vi "Read_Write_ADAM_setup.vi"(3 "Mode":T1(ring)) -> ()   [LabVIEW 2010]
uses:
  ADAM Client/Sub VIs/ADAM Controls/Channel_State.ctl
  Anemometry/Anemometry Sub Vis/Globals/Constants_global.vi
  Anemometry/Anemometry Sub Vis/Globals/Gas_management_global.vi
  Exp conditions/EnFlo_Tun_Setup_global.vi
  ADAM_Global.vi
  Channel_Description_Global.vi
panel:
  out "Setup Filename":string
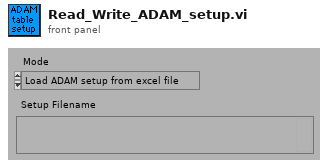
[diagram p1: front panel]
types:
  T1 = enum16{"Load ADAM setup from excel file", "Save ADAM setup to excel file"}
  T2 = typedef "Channel_State.ctl" = enum16{"On", "Off", "Always On", "Always Off"}
  T3 = typedef "Ch_description_ADAM.ctl" = cluster{"Ch Name":string, "Type":T4, "Function":T5, "Ch State":T2, "Calibration type":T6, "A":dbl, "B":dbl, "C":dbl, "D":dbl, "Comments":string, "Address":T7, "String":string, "Duty":u16}
  T4 = typedef "Module_type_ADAM.ctl" = enum16{"4011", "4012", "4013", "4014", "4016", "4017", "4018", "4021", "4050", "4052", "4053", "4060", "4080", "5000", "5017", "5018", "5024", "5051", "5056", "5060", "6060", "Tracker", "WEST", "GILL", "JEM", "VICI", "Vaisala", "DRUCK", "Run VI Named:", "IR2100", "PPT", "Comparator", "VIRTUAL", "Hold Value", "Read A", "Read Ch", "Coded", "Client Info", "Web Client", "X10", "Test"}
  T5 = typedef "Function_ADAM.ctl" = enum16{"Analogue Input", "Digital Input", "Event counter", "Event rate", "Analogue Output", "Digital Output", "Relay Output"}
  T6 = typedef "Calib_type_ADAM.ctl" = enum16{"Raw", "Bx + A", "Cx^2 + Bx + A", "Dx^3 + Cx^2 + Bx + A", "In Band", "Hi-Tec Q", "Hi-Tec M_dot", "Text"}
  T7 = typedef "Address.ctl" = cluster{"Main":i32, "Ch.":i32, "Sub":i32, "Port Name":string}
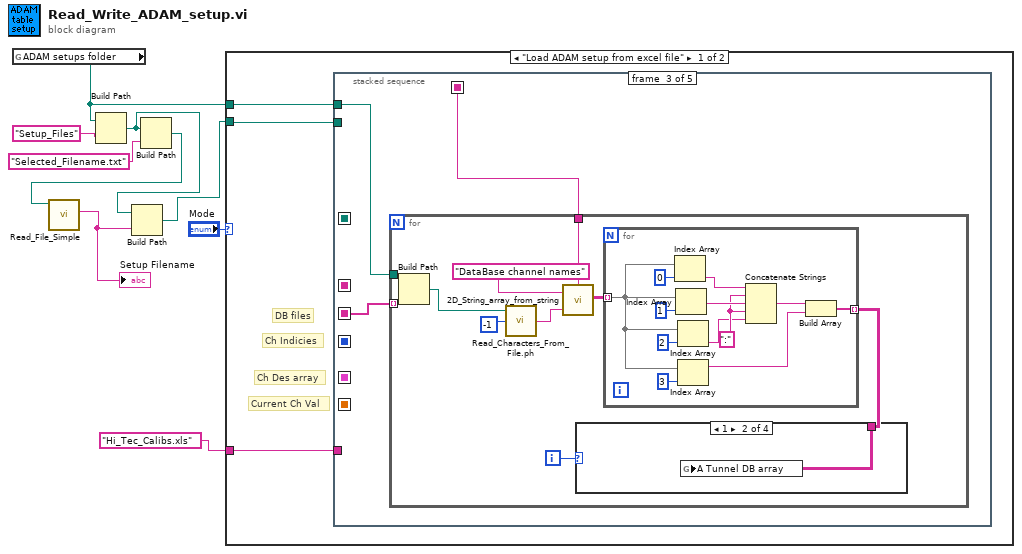
[diagram p0: block diagram]
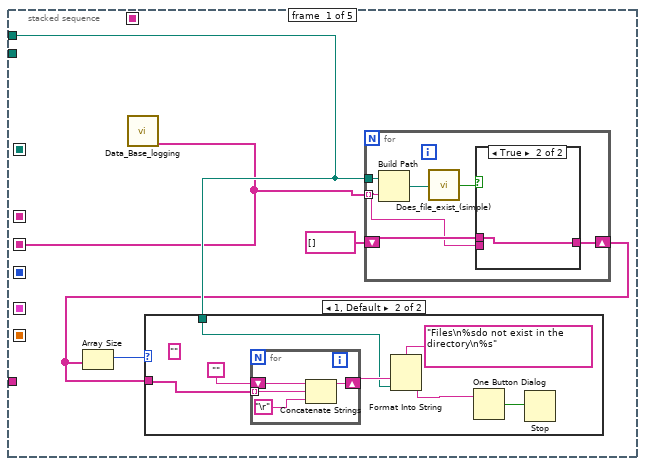
[diagram p2: hidden frame]
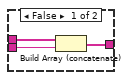
[diagram p4: hidden frame]
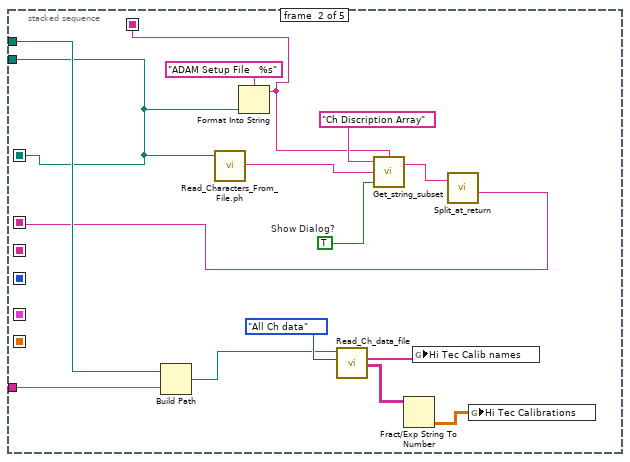
[diagram p5: hidden frame]
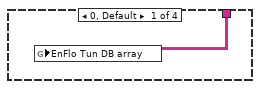
[diagram p6: hidden frame]
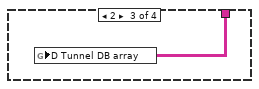
[diagram p7: hidden frame]
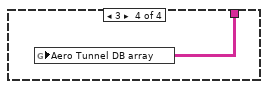
[diagram p8: hidden frame]
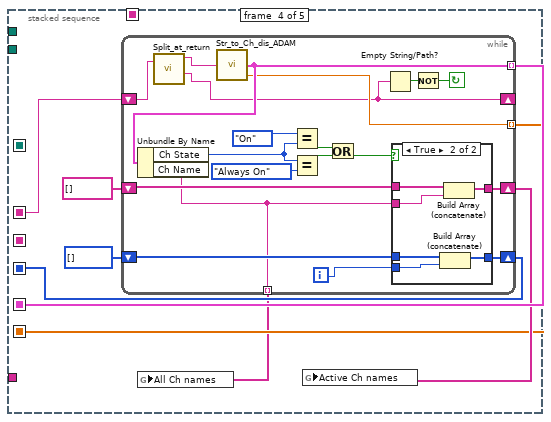
[diagram p9: hidden frame]
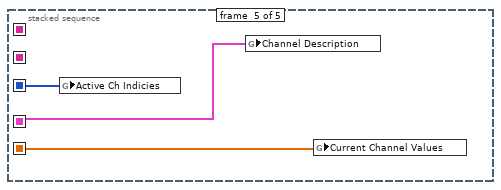
[diagram p11: hidden frame]
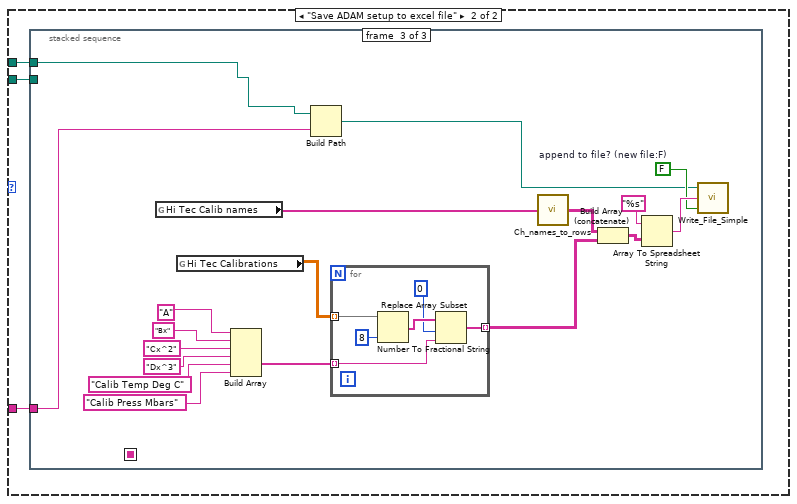
[diagram p12: hidden frame]
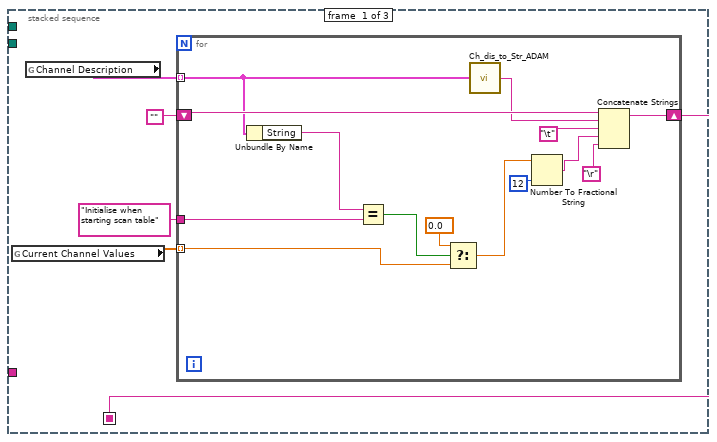
[diagram p13: hidden frame]
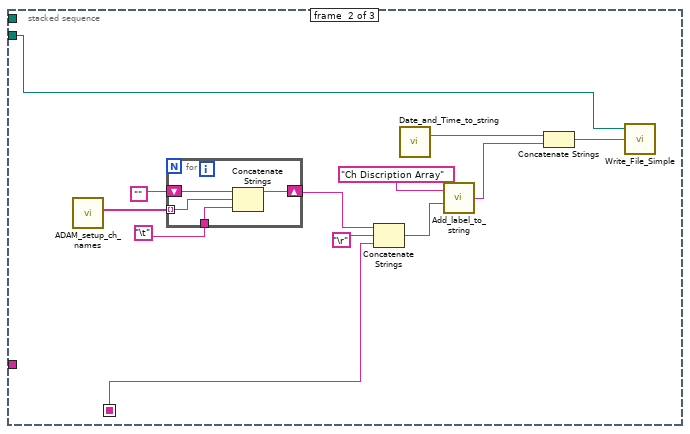
[diagram p14: hidden frame]
diagram:
  n1 = global read "Constants_global.vi" "ADAM setups folder"() -> (w8:path)
  n2 = Build Path(base path=w8, name or relative path="Setup_Files") -> (appended path=w4:path)
  n3 = Build Path(base path=w4, name or relative path="Selected_Filename.txt" ("Substring")) -> (appended path=w5:path)
  n4 = call "Read_File_Simple.vi"("Filename"=w5) -> ("string"=w3:string)  [unwired: 2 in, 7 out]
  "Setup Filename" <- w3
  n5 = Build Path(base path=w4, name or relative path=w3) -> (appended path=w2:path)
  n6 = case shown="\"Load ADAM setup from excel file\"" "Mode" {
    tunnel: w2 -> [w12 w123]
    tunnel: w8 -> [w11 w122]
    tunnel: "Hi_Tec_Calibs.xls" ("name or relative path") -> [w10 w121]
    frame "Load ADAM setup from excel file" {
      # "DB files"
      # "Ch Indicies"
      # "Current Ch Val"
      # "Ch Des array"
      n7 = stacked-sequence {
        seq-local: [_ w42 _ _ _] -> [_ _ _ w90 _]
        seq-local: [_ _ _ w89 _] -> [_ _ _ _ w118]
        seq-local: [_ _ _ w84 _] -> [_ _ _ _ w119]
        seq-local: [_ _ _ w85 _] -> [_ _ _ _ w120]
        seq-local: [_ w40 _ _ _] -> [_ _ _ _ _]
        seq-local: [w13 _ _ _ _] -> [_ _ w55 _ _]
        seq-local: [_ w39 _ _ _] -> [_ _ w54 _ _]
        tunnel: w12 -> [_ w40 _ _ _]
        tunnel: w11 -> [w15 w47 w56 _ _]
        tunnel: w10 -> [_ w44 _ _ _]
        frame #0 {
          n8 = call "Data_Base_logging.vi"() -> ("DB Setup files"=w13:string[])  [unwired: 4 out]
          n9 = for {
            tunnel: w13 -> [w30] mode=indexing
            tunnel: w15 -> [w34]
            shift-right: [w29] -> w14
            shift-left: string[] [] -> [w31]
            n10 = Build Path(base path=w34, name or relative path=w30) -> (appended path=w33:path)
            n11 = call "Does_file_exist_(simple).vi"("Pathname"=w33) -> ("exists?"=w32:bool)
            n12 = case shown="True" w32 {
              tunnel: w31 -> [w37 w38]
              tunnel: w30 -> [w36 _]
              tunnel: [w35 w38] -> w29
              frame False {
                n13 = Build Array (concatenate)(w37, w36) -> (w35:string[])
              }
              frame True {
              }
            }
          }
          n14 = Array Size(array=w14) -> (size(s)=w16:i32)
          n15 = case shown="1, Default" w16 {
            tunnel: w15 -> [_ w21]
            tunnel: w14 -> [_ w23]
            frame 0 {
            }
            frame 1, Default {
              (unwired) ""
              n16 = for {
                shift-right: [w25] -> w22
                shift-left: "" -> [w28]
                tunnel: w23 -> [w26] mode=indexing
                n17 = Concatenate Strings(w28, w26, "\r") -> (w25:string)
              }
              n18 = Format Into String(format string="Files\n%sdo not exist in the directory\n%s" ("Format String"), w22, w21) -> (resulting string=w19:string)  [unwired: 2 in, 1 out]
              n19 = One Button Dialog(message=w19) -> (true=w18:bool)  [unwired: 1 out]
              n20 = Stop(stop? (T)=w18) -> ()
            }
          }
        }
        frame #1 {
          w48 = TRUE  # Show Dialog?
          n21 = Build Path(base path=w47, name or relative path=w44) -> (appended path=w46:path)
          n22 = call "Read_Characters_From_File.ph.vi"("file path (dialog if empty)"=w40) -> ("character string"=w45:string)  [unwired: 1 in, 7 out]
          n23 = Format Into String(format string="ADAM Setup File   %s", w40) -> (resulting string=w39:string)  [unwired: 2 in, 1 out]
          n24 = call "Read_Ch_data_file.vi"("Output"=enum16{"All Ch data", "The last few rows"}."All Ch data", "Filename"=w46) -> ("Channel Values"=w50:string[][], "Merged Channels"=w51:string[])  [unwired: 3 in, 3 out]
          n25 = call "Get_string_subset.vi"("String Name"=w39, "Show Dialog?"=w48, "String to split"=w45, "File Label"="Ch Discription Array") -> ("Output string"=w43:string)  [unwired: 1 out]
          n26 = Fract/Exp String To Number(string=w50) -> (number=w49:dbl[][])  [unwired: 4 out]
          n27 = global write "Gas_management_global.vi" "Hi Tec Calib names"(w51) -> ()
          n28 = call "Split_at_return.vi"("String"=w43) -> ("after substring"=w42:string)  [unwired: 1 in, 3 out]
          n29 = global write "Gas_management_global.vi" "Hi Tec Calibrations"(w49) -> ()
        }
        frame #2 {
          n30 = for {
            tunnel: w56 -> [w60]
            tunnel: w55 -> [w59] mode=indexing
            tunnel: w54 -> [w57]
            i -> [w62]
            n31 = Build Path(base path=w60, name or relative path=w59) -> (appended path=w58:path)
            n32 = call "Read_Characters_From_File.ph.vi"("file path (dialog if empty)"=w58, "number of characters (all:-1)"=-1) -> ("character string"=w63:string)  [unwired: 7 out]
            n33 = call "2D_String_array_from_string.vi"("String Name"=w57, "Input string"=w63, "Array title"="DataBase channel names") -> ("2D data array"=w64:string[][])
            n34 = for {
              tunnel: w64 -> [w74] mode=indexing
              tunnel: [w72] -> w61 mode=indexing
              w77 = ":"
              n35 = Index Array(array=w74, index=0) -> (element=w79:string)
              n36 = Index Array(array=w74, index=1) -> (element=w78:string)
              n37 = Index Array(array=w74, index=2) -> (element=w76:string)
              n38 = Index Array(array=w74, index=3) -> (element=w73:string)
              n39 = Concatenate Strings(w79, w77, w78, w77, w76) -> (w71:string)
              n40 = Build Array(w71, w73) -> (w72:string[])
            }
            n41 = case shown="1" w62 {
              tunnel: w61 -> [w67 w68 w69 w70]
              frame 0, Default {
                n42 = global write "EnFlo_Tun_Setup_global.vi" "EnFlo Tun DB array"(w67) -> ()
              }
              frame 1 {
                n43 = global write "EnFlo_Tun_Setup_global.vi" "A Tunnel DB array"(w68) -> ()
              }
              frame 2 {
                n44 = global write "EnFlo_Tun_Setup_global.vi" "D Tunnel DB array"(w69) -> ()
              }
              frame 3 {
                n45 = global write "EnFlo_Tun_Setup_global.vi" "Aero Tunnel DB array"(w70) -> ()
              }
            }
          }
        }
        frame #3 {
          n46 = while {
            tunnel: [w94] -> w83 mode=indexing
            tunnel: [w95] -> w84 mode=indexing
            shift-left: i32[] [] -> [w103]
            shift-right: [w104] -> w85
            shift-left: string[] [] -> [w106]
            shift-right: [w105] -> w88
            tunnel: [w107] -> w89 mode=indexing
            shift-left: w90 -> [w91]
            shift-right: [w93] -> _
            i -> [w102]
            stop <- w108 continue-if-true
            n47 = call "Split_at_return.vi"("String"=w91) -> ("before substring"=w92:string, "after substring"=w93:string)  [unwired: 1 in, 2 out]
            n48 = call "Str_to_Ch_dis_ADAM.vi"("String Row"=w92) -> ("Value"=w95:dbl, "Ch Description"=w107:T3)  [unwired: 1 in, 2 out]
            n49 = Unbundle By Name(w107) -> ("Ch State"=w97:T2, "Ch Name"=w94:string)
            n50 = Equal?(x=Channel_State."On" ("Channel State"), y=w97) -> (x = y?=w99:bool)
            n51 = Equal?(x=w97, y=Channel_State."Always On" ("Channel State")) -> (x = y?=w98:bool)
            n52 = Or(x=w99, y=w98) -> (x .or. y?=w96:bool)
            n53 = Empty String/Path?(string/path=w93) -> (empty?=w109:bool)
            n54 = case shown="True" w96 {
              tunnel: w94 -> [_ w117]
              tunnel: w106 -> [w111 w116]
              tunnel: [w111 w115] -> w105
              tunnel: w103 -> [w110 w112]
              tunnel: w102 -> [_ w113]
              tunnel: [w110 w114] -> w104
              frame False {
              }
              frame True {
                n55 = Build Array (concatenate)(w112, w113) -> (w114:i32[])
                n56 = Build Array (concatenate)(w116, w117) -> (w115:string[])
              }
            }
            n57 = Not(x=w109) -> (.not. x?=w108:bool)
          }
          n58 = global write "ADAM_Global.vi" "All Ch names"(w83) -> ()
          n59 = global write "ADAM_Global.vi" "Active Ch names"(w88) -> ()
        }
        frame #4 {
          n60 = global write "ADAM_Global.vi" "Active Ch Indicies"(w120) -> ()
          n61 = global write "Channel_Description_Global.vi" "Channel Description"(w118) -> ()
          n62 = global write "ADAM_Global.vi" "Current Channel Values"(w119) -> ()
        }
      }
    }
    frame "Save ADAM setup to excel file" {
      n63 = stacked-sequence {
        seq-local: [w127 _ _] -> [_ w147 _]
        tunnel: w123 -> [_ w144 _]
        tunnel: w122 -> [_ _ w168]
        tunnel: w121 -> [_ _ w167]
        frame #0 {
          n64 = global read "ADAM_Global.vi" "Current Channel Values"() -> (w126:dbl[])
          n65 = global read "Channel_Description_Global.vi" "Channel Description"() -> (w124:T3[])
          n66 = for {
            shift-right: [w129] -> w127
            shift-left: "" -> [w142]
            tunnel: w124 -> [w141] mode=indexing
            tunnel: w126 -> [w140] mode=indexing
            tunnel: "Initialise when starting scan table" ("y") -> [w139]
            n67 = Unbundle By Name(w141) -> ("String"=w132:string)
            n68 = Equal?(x=w132, y=w139) -> (x = y?=w131:bool)
            n69 = Select(t=0.0, s=w131, f=w140) -> (s? t:f=w133:dbl)
            n70 = call "Ch_dis_to_Str_ADAM.vi"("Ch Description"=w141) -> ("String Row"=w138:string)  [unwired: 4 out]
            n71 = Number To Fractional String(number=w133, precision (6)=i16 12) -> (F-format string=w134:string)  [unwired: 2 out]
            n72 = Concatenate Strings(w142, w138, "\t", w134, "\r") -> (w129:string)
          }
        }
        frame #1 {
          n73 = call "ADAM_setup_ch_names.vi"() -> ("Ch Names"=w146:string[])  [unwired: 1 out]
          n74 = for {
            shift-right: [w155] -> w145
            shift-left: "" -> [w158]
            tunnel: "\t" -> [w156]
            tunnel: w146 -> [w157] mode=indexing
            n75 = Concatenate Strings(w158, w157, w156) -> (w155:string)
          }
          n76 = Concatenate Strings(w145, "\r", w147) -> (w153:string)
          n77 = call "Date_and_Time_to_string.vi"() -> ("Date and time (spreadsheet)"=w152:string)
          n78 = call "Add_label_to_string.vi"("String to write"=w153, "File Label"="Ch Discription Array") -> ("Output string"=w151:string)
          n79 = Concatenate Strings(w152, w151) -> (w143:string)
          n80 = call "Write_File_Simple.vi"("character string"=w143, "file path"=w144) -> ()  [unwired: 1 in, 2 out]
        }
        frame #2 {
          w162 = FALSE  # append to file? (new file:F)
          n81 = global read "Gas_management_global.vi" "Hi Tec Calib names"() -> (w160:string[])
          n82 = global read "Gas_management_global.vi" "Hi Tec Calibrations"() -> (w176:dbl[][])
          n83 = Build Array("A", "Bx", "Cx^2", "Dx^3", "Calib Temp Deg C", "Calib Press Mbars") -> (w169:string[])
          n84 = Build Path(base path=w168, name or relative path=w167) -> (appended path=w161:path)
          n85 = for {
            tunnel: w176 -> [w182] mode=indexing
            tunnel: [w179] -> w159 mode=indexing
            tunnel: w169 -> [w177] mode=indexing
            n86 = Number To Fractional String(number=w182, precision (6)=i16 8) -> (F-format string=w180:string[])  [unwired: 2 out]
            n87 = Replace Array Subset(array=w180, new element=w177, index=0) -> (w179:string[])
          }
          n88 = call "Ch_names_to_rows.vi"("Channel Names"=w160) -> ("3 Row names"=w166:string[][])
          n89 = Build Array (concatenate)(w166, w159) -> (w164:string[][])
          n90 = Array To Spreadsheet String(array=w164, 3:"%s" ("format string")) -> (spreadsheet string=w163:string)  [unwired: 1 out]
          n91 = call "Write_File_Simple.vi"("append to file? (new file:F)"=w162, "character string"=w163, "file path"=w161) -> ()  [unwired: 2 out]
        }
      }
    }
  }
